vi "Bisection Test.vi"() -> ()   [LabVIEW 2010]
uses:
  <vilib>/Analysis/Matrix/Datatypes/RealMatrix.ctl
  <vilib>/Analysis/Matrix/NI_Matrix.lvlib
  Subsystems/Global Variables.vi
panel:
  in  "Deform Array":dbl[](array[numeric])=[1.0, 1.0, 1.0, 0.0, 0.0, 0.0, 0.0, 0.0, 0.0]
  out "Assign Pt OOB":bool
  out "Assign Pt*":dbl[](array[numeric])
  in  "Assign Pt":dbl[](array[numeric])=[0.0, 5.0, 0.0]
  in  "Current Pt":dbl[](array[numeric])=[0.0, 0.0, 0.0]
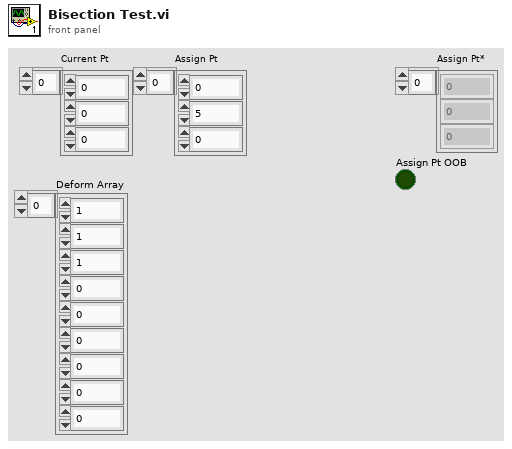
[diagram p1: front panel]
types:
  T1 = typedef "NI_Matrix.lvlib/RealMatrix.ctl" = dbl[][]
  T2 = cluster{"X Grid":dbl[], "Y Grid":dbl[], "Za_true Surf":dbl[][], "Iris Center":dbl[], "Zp_true Surf":dbl[][], "Pinv":T1, "za_true":dbl, "za_work":dbl, "zp_work":dbl, "zp_true":dbl}
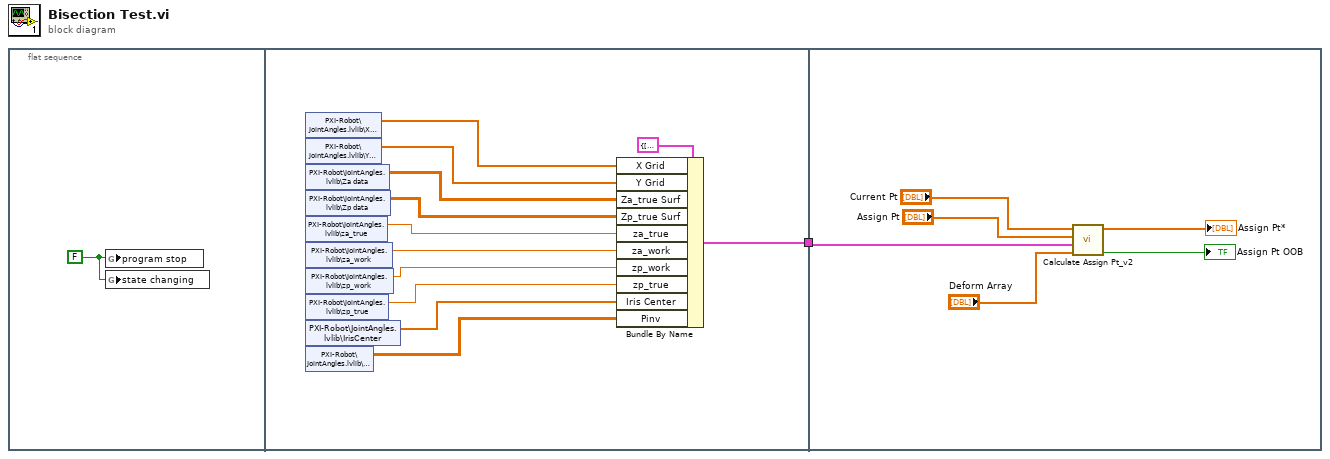
[diagram p0: block diagram]
diagram:
  n1 = flat-sequence {
    tunnel: [w3] -> w1
    tunnel: w1 -> [w16]
    frame #0 {
      w2 = FALSE ("program stop")
      n2 = global write "Global Variables.vi" "program stop"(w2) -> ()
      n3 = global write "Global Variables.vi" "state changing"(w2) -> ()
    }
    frame #1 {
      n4 = shared-variable "PXI-Robot\\JointAngles.lvlib\\X grid"() -> (w14:dbl[])  [unwired: 1 in, 1 out]
      n5 = shared-variable "PXI-Robot\\JointAngles.lvlib\\Y grid"() -> (w13:dbl[])  [unwired: 1 in, 1 out]
      n6 = shared-variable "PXI-Robot\\JointAngles.lvlib\\Za data"() -> (w12:dbl[][])  [unwired: 1 in, 1 out]
      n7 = shared-variable "PXI-Robot\\JointAngles.lvlib\\Zp data"() -> (w10:dbl[][])  [unwired: 1 in, 1 out]
      n8 = shared-variable "PXI-Robot\\JointAngles.lvlib\\za_true"() -> (w4:dbl)  [unwired: 1 in, 1 out]
      n9 = shared-variable "PXI-Robot\\JointAngles.lvlib\\za_work"() -> (w5:dbl)  [unwired: 1 in, 1 out]
      n10 = shared-variable "PXI-Robot\\JointAngles.lvlib\\zp_work"() -> (w6:dbl)  [unwired: 1 in, 1 out]
      n11 = shared-variable "PXI-Robot\\JointAngles.lvlib\\zp_true"() -> (w7:dbl)  [unwired: 1 in, 1 out]
      n12 = shared-variable "PXI-Robot\\JointAngles.lvlib\\IrisCenter"() -> (w9:dbl[])  [unwired: 1 in, 1 out]
      n13 = shared-variable "PXI-Robot\\JointAngles.lvlib\\Pinv"() -> (w8:T1)  [unwired: 1 in, 1 out]
      n14 = Bundle By Name(cluster=T2 {"X Grid"=[], "Y Grid"=[], "Za_true Surf"=[], "Iris Center"=[], "Zp_true Surf"=[], "Pinv"=[], "za_true"=0.0, "za_work"=0.0, "zp_work"=0.0, "zp_true"=0.0} ("Eye Model Cluster"), "X Grid"=w14, "Y Grid"=w13, "Za_true Surf"=w12, "Zp_true Surf"=w10, "za_true"=w4, "za_work"=w5, "zp_work"=w6, "zp_true"=w7, "Iris Center"=w9, "Pinv"=w8) -> (w3:T2)
    }
    frame #2 {
      n15 = call "Calculate Assign Pt_v2.vi"("Deform Array"="Deform Array", "Eye Model Cluster"=w16, "Assign Pt"="Assign Pt", "Current Pt"="Current Pt") -> ("Assign Pt OOB"=→"Assign Pt OOB":bool, "Assign Pt*"=→"Assign Pt*":dbl[])  [unwired: 6 in]
    }
  }
